vi "PRL TS Round to Nearest 10ms.vi"(11 "Time Stamp In":timestamp) -> (3 "Time Stamp Out":timestamp)   [LabVIEW 2018, in "S3DK.lvlib" / "PMU Recorder Light.lvlib"]
uses:
  PMU Recorder Light.lvlib
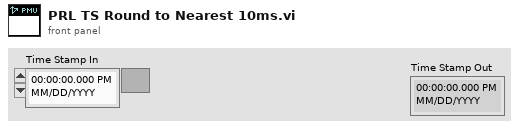
[diagram p1: front panel]
types:
  T1 = typedef "LVDateTimeRec.ctl" = cluster{"fractional second":dbl, "second":i32, "minute":i32, "hour":i32, "day of month":i32, "month":i32, "year":i32, "day of week":i32, "day of year":i32, "DST":i32}
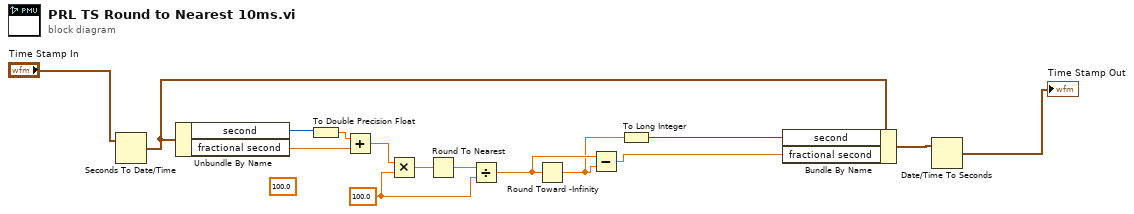
[diagram p0: block diagram]
diagram:
  (unwired) 100.0 ("y")
  w12 = 100.0 ("y")
  n1 = Seconds To Date/Time(time stamp (now)="Time Stamp In") -> (date time rec=w11:T1)  [unwired: 1 in]
  n2 = Unbundle By Name(w11) -> ("second"=w8:i32, "fractional second"=w6:dbl)
  n3 = To Double Precision Float(number=w8) -> (double precision float=w7:dbl)
  n4 = Add(x=w7, y=w6) -> (x+y=w5:dbl)
  n5 = Multiply(x=w5, y=w12) -> (x*y=w14:dbl)
  n6 = Round To Nearest(number=w14) -> (nearest integer value=w13:dbl)
  n7 = Divide(x=w13, y=w12) -> (x/y=w4:dbl)
  n8 = Round Toward -Infinity(1:w4) -> (0:w2:dbl)
  n9 = Subtract(x=w4, y=w2) -> (x-y=w1:dbl)
  n10 = To Long Integer(number=w2) -> (32bit integer=w3:i32)
  n11 = Bundle By Name(cluster=w11, "second"=w3, "fractional second"=w1) -> (w10:T1)
  n12 = Date/Time To Seconds(2:w10) -> (0:→"Time Stamp Out":timestamp)  [unwired: 1 in]
